vi "Flow cell controller globals.vi"() -> ()   [LabVIEW 2015]
panel:
  in  "Flow Rate":dbl=100.0
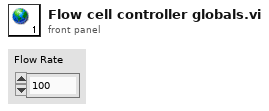
[diagram p1: front panel]
diagram:
